vi "Solenoid Shooter Control.vi"(11 "Shoot Button":bool) -> (3 "Solenoid Value":T1)   [LabVIEW 2012]
uses:
  <vilib>/Rock Robotics/WPI/Solenoid/WPI_SolenoidValue.ctl
  MAIN ROBOT/Robot Global Data.vi
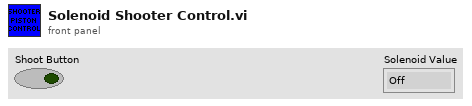
[diagram p1: front panel]
types:
  T1 = typedef "WPI_SolenoidValue.ctl" = enum16{"Off", "On", "Forward", "Reverse"}
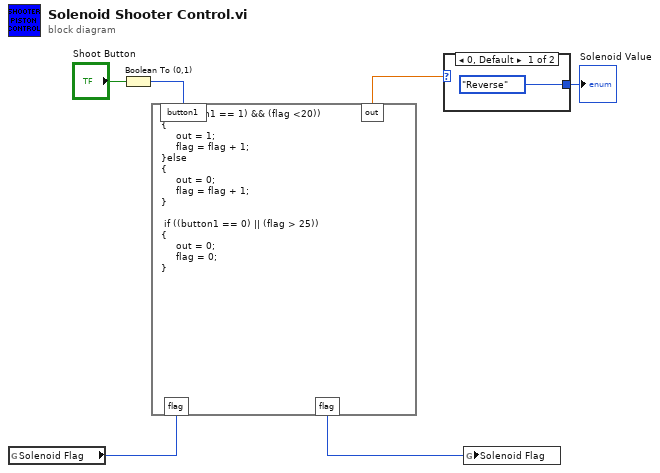
[diagram p0: block diagram]
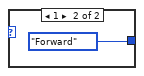
[diagram p2: hidden frame]
diagram:
  n1 = global read "Robot Global Data.vi" "Solenoid Flag"() -> (w5:i8)
  n2 = Boolean To (0,1)(Boolean="Shoot Button") -> (0, 1=w2:i16)
  n3 = formula code="if ((button1 == 1) && (flag <20))\n{\n     out = 1;\n     flag = flag + 1;\n}else\n{\n     out = 0;\n     flag = flag + 1;\n}\n\n if ((button1 == 0) || (flag > 25))\n{\n     out = 0;\n     flag = 0;\n}"("button1"=w2, "flag"=w5) -> ("out"=w1:dbl, "flag"=w6:i8)
  n4 = case shown="0, Default" w1 {
    tunnel: [WPI_SolenoidValue."Reverse" ("Value") WPI_SolenoidValue."Forward" ("Value")] -> w3
    frame 0, Default {
    }
    frame 1 {
    }
  }
  "Solenoid Value" <- w3
  n5 = global write "Robot Global Data.vi" "Solenoid Flag"(w6) -> ()
